vi "generate_DAC_voltages_V3_justFPGATrajectory.vi"(7 "focus mode?":bool, 8 "derived values":T1, 9 "scan specification":T4={"x amplitude"=0, "x resolution (pixels)"=0, "x offset fly-forward (iterations)"=0, "x offset fly-back (iterations)"=0, "y resolution (nr. of lines)"=0, "y step size"=0, "iterations per pixel"=0, "number of frames"=0, "y offset (pixels)"=0, "number of y-brake lines  (before y-fly-back)"=0, "number y-brake lines (after y-fly-back)"=0, "number of y-fly-back steps"=8, "lines per z step"=0, "number of z/intensity tuples"=0, "number of repetitions (volumes or planes)"=0, "z step size derived"=0, "choose the beginning of z scan"=FALSE, "number of frames (settings)"=0, "FPGA trajectory?"=FALSE}, 10 "counter cluster in":T2, 11 "resonant trigger":bool) -> (0 "acquire?":bool, 1 "fly-back acquisition phase?":bool, 2 "counter cluster out":T2, 3 "DAC voltages":T3 {"ch6" max=4095 step=1; "ch5" max=4095 step=1; "ch4" max=4095 step=1; "ch3" max=4095 step=1; "ch2" max=4095 step=1; "ch1" max=4095 step=1; "ch0" max=4095 step=1})   [LabVIEW 2010]
uses:
  scan_specification_cluster.ctl
  common_typedefs/DAC_voltage_cluster.ctl
  counter_cluster.ctl
  derived_values_cluster.ctl
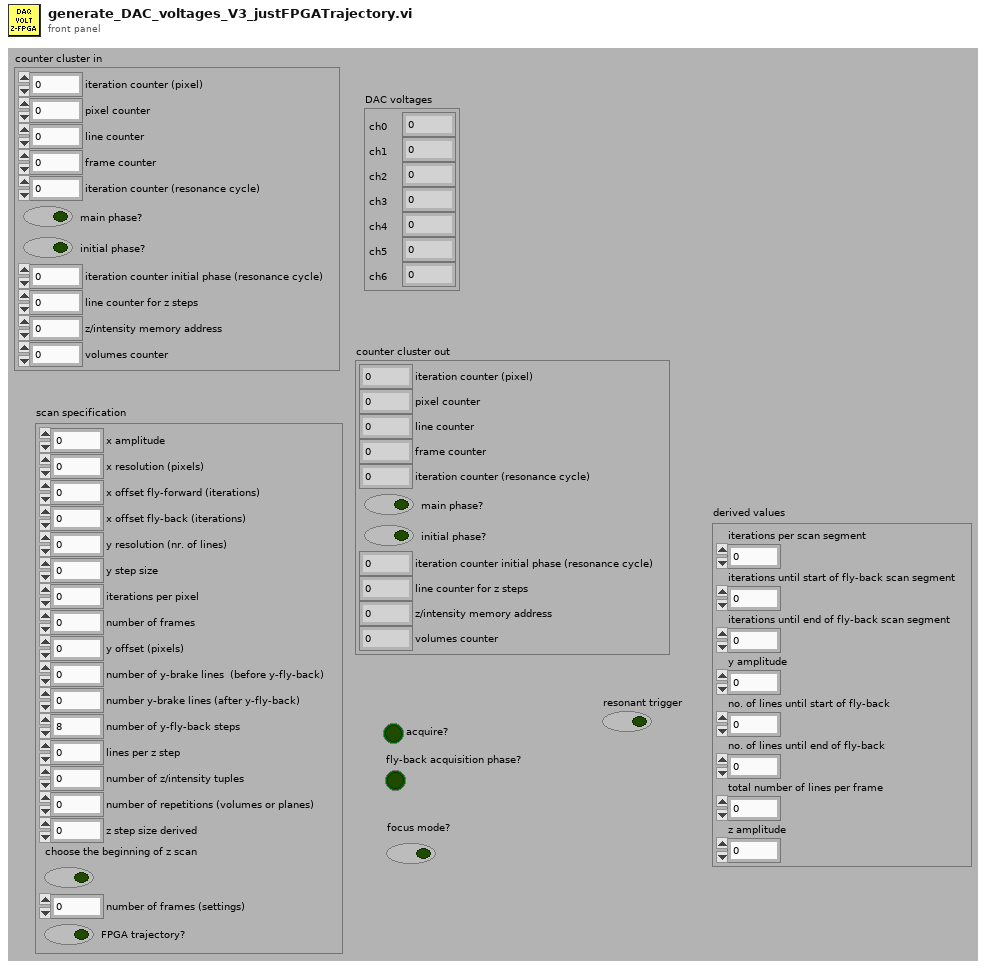
[diagram p1: front panel]
types:
  T1 = typedef "derived_values_cluster.ctl" = cluster{"iterations per scan segment":u16, "iterations until start of fly-back scan segment":u16, "iterations until end of fly-back scan segment":u16, "y amplitude":u16, "no. of lines until start of fly-back":u16, "no. of lines until end of fly-back":u16, "total number of lines per frame ":u16, "z amplitude":u16}
  T2 = typedef "counter_cluster.ctl" = cluster{"iteration counter (pixel)":u16, "pixel counter":u16, "line counter":u16, "frame counter":u16, "iteration counter (resonance cycle)":u16, "main phase?":bool, "initial phase?":bool, "iteration counter initial phase (resonance cycle)":u16, "line counter for z steps":u16, "z/intensity memory address":u32, "volumes counter":u16}
  T3 = typedef "DAC_voltage_cluster.ctl" = cluster{"ch0":u16, "ch1":i16, "ch2":i16, "ch3":u16, "ch4":u16, "ch5":u16, "ch6":u16}
  T4 = typedef "scan_specification_cluster.ctl" = cluster{"x amplitude":u16, "x resolution (pixels)":u16, "x offset fly-forward (iterations)":u16, "x offset fly-back (iterations)":u16, "y resolution (nr. of lines)":u16, "y step size":u16, "iterations per pixel":u16, "number of frames":i32, "y offset (pixels)":u16, "number of y-brake lines  (before y-fly-back)":u16, "number y-brake lines (after y-fly-back)":u16, "number of y-fly-back steps":u16, "lines per z step":u16, "number of z/intensity tuples":u16, "number of repetitions (volumes or planes)":i32, "z step size derived":u16, "choose the beginning of z scan":bool, "number of frames (settings)":i32, "FPGA trajectory?":bool}
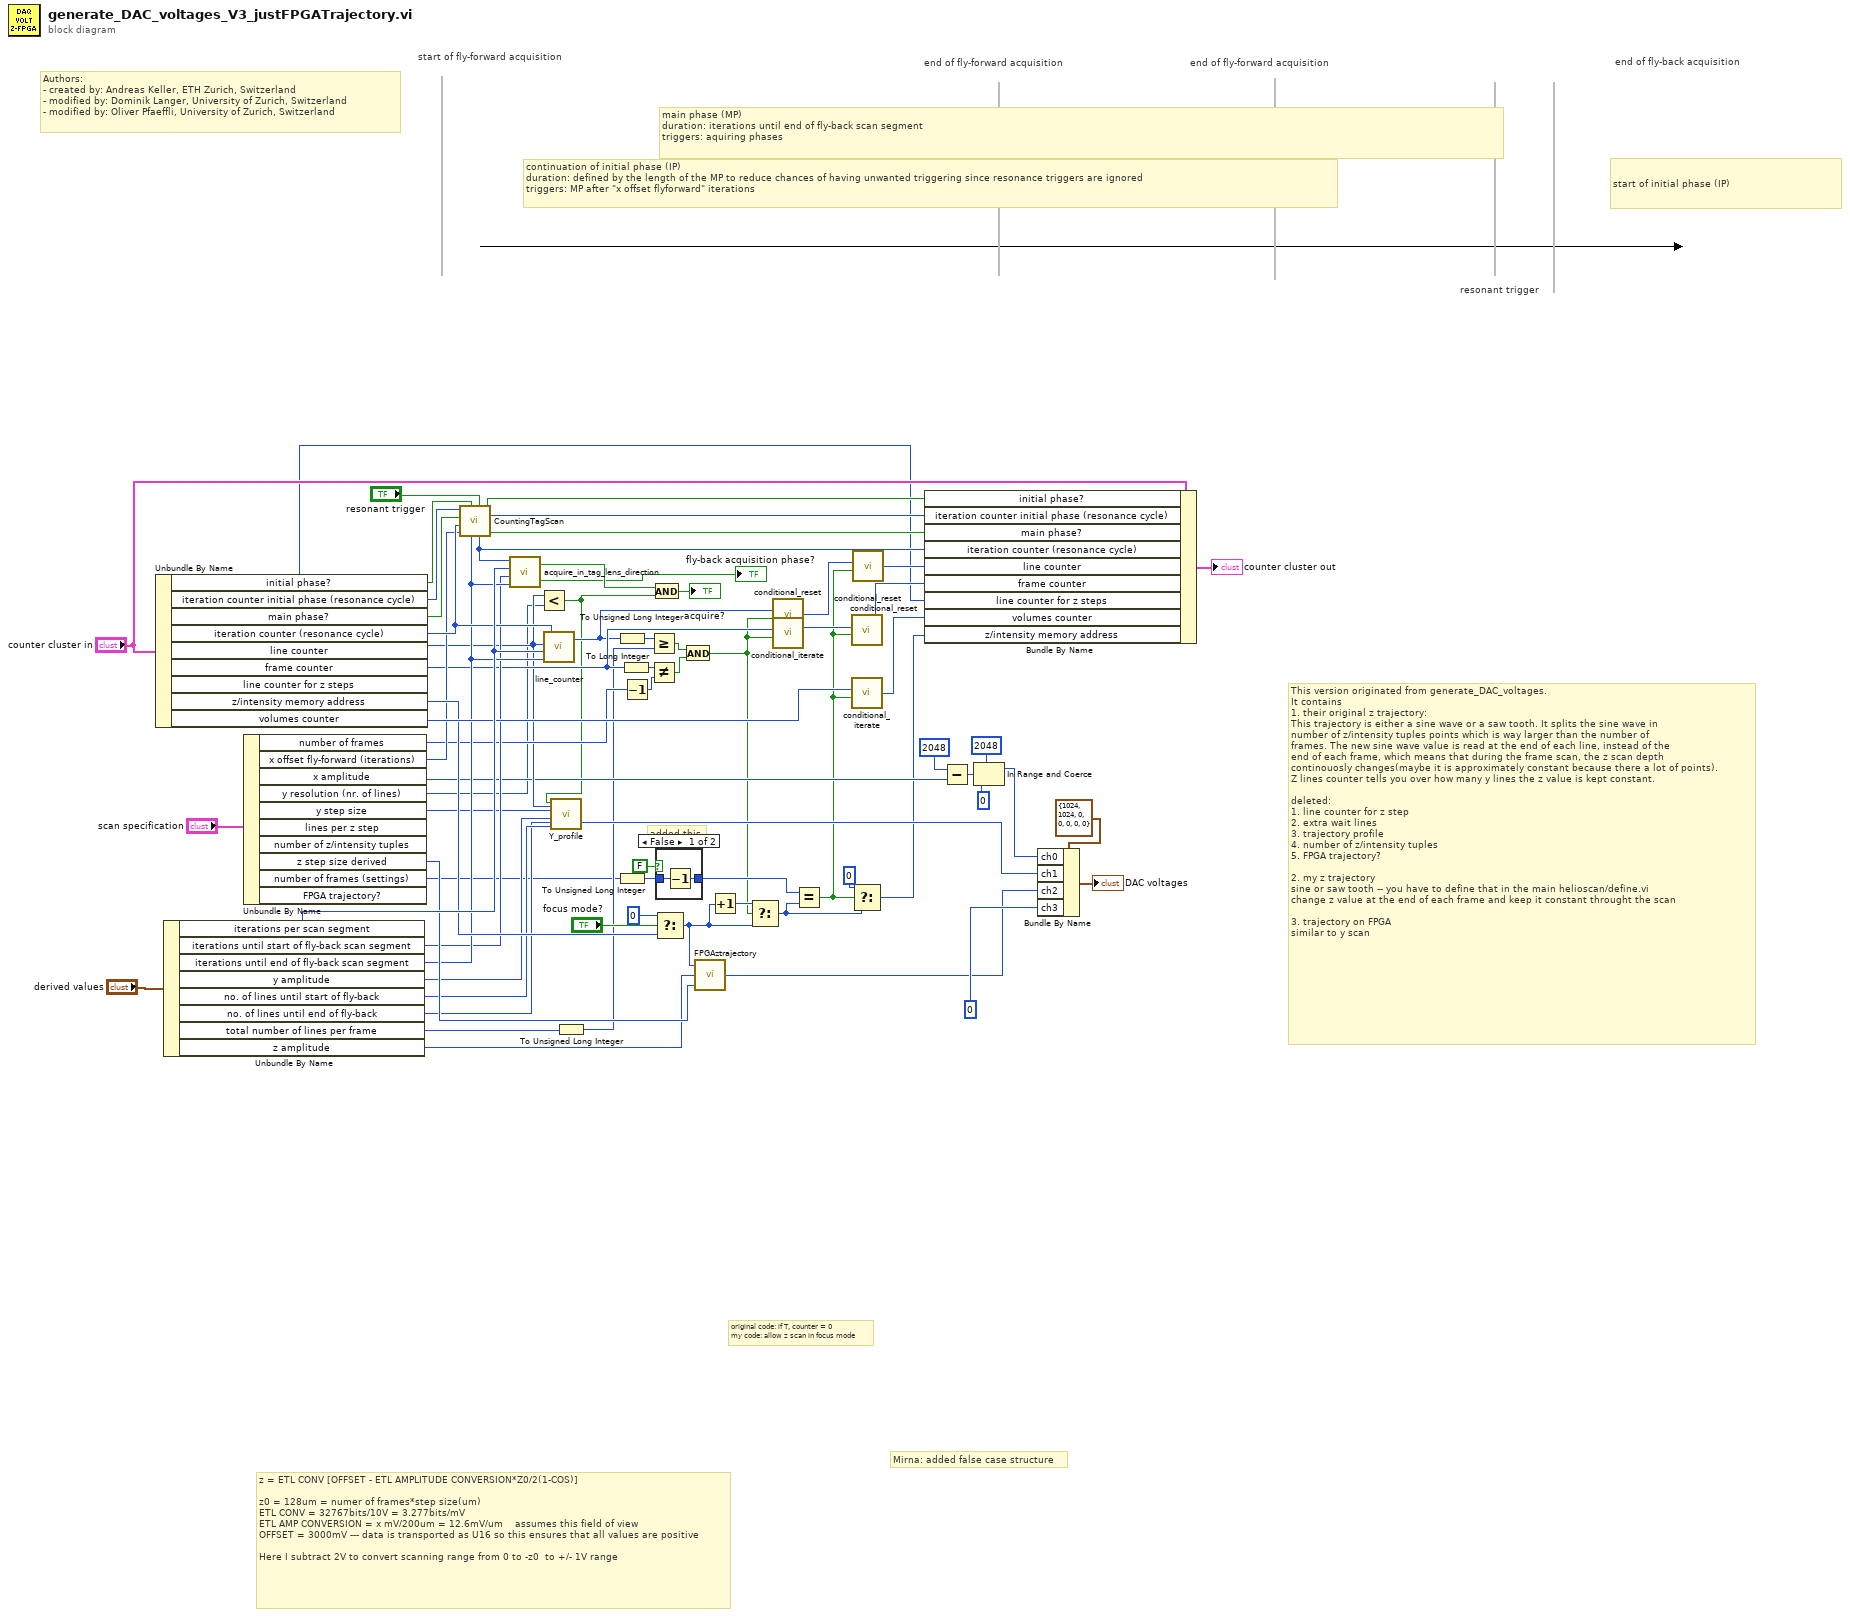
[diagram p0: block diagram]
diagram:
  # "This version originated from generate_DAC_voltages.\nIt contains \n1. their original z trajectory:\nThis trajectory is either a sine wave or a saw tooth. It splits the sine wave in\nnumber of z/intensity tuples points which is way larger than the number of\nframes. The new sine wave value is read at the end of each line, instead of the\nend of each frame, which means that during the frame scan, the z scan depth \ncontinouosly changes(maybe it is approximately constant because there a lot of points).\nZ lines counter tells you over how many y lines the z value is kept constant.\n\ndeleted: \n1. line counter for z step\n2. extra wait lines\n3. trajectory profile\n4. number of z/intensity tuples\n5. FPGA trajectory?\n\n2. my z trajectory\nsine or saw tooth -- you have to define that in the main helioscan/define.vi\nchange z value at the end of each frame and keep it constant throught the scan\n\n3. trajectory on FPGA\nsimilar to y scan"
  # "added this"
  # "z = ETL CONV [OFFSET - ETL AMPLITUDE CONVERSION*Z0/2(1-COS)]\n\nz0 = 128um = numer of frames*step size(um)\nETL CONV = 32767bits/10V = 3.277bits/mV\nETL AMP CONVERSION = x mV/200um = 12.6mV/um    assumes this field of view\nOFFSET = 3000mV --- data is transported as U16 so this ensures that all values are positive\n\nHere I subtract 2V to convert scanning range from 0 to -z0  to +/- 1V range"
  # "original code: if T, counter = 0\nmy code: allow z scan in focus mode"
  # "Mirna: added false case structure"
  # "start of initial phase (IP)"
  # "continuation of initial phase (IP)\nduration: defined by the length of the MP to reduce chances of having unwanted triggering since resonance triggers are ignored\ntriggers: MP after \"x offset flyforward\" iterations"
  # "end of fly-back acquisition"
  # "end of fly-forward acquisition"
  # "end of fly-forward acquisition"
  # "start of fly-forward acquisition"
  # "main phase (MP)\nduration: iterations until end of fly-back scan segment\ntriggers: aquiring phases"
  # "resonant trigger"
  # "Authors: \n- created by: Andreas Keller, ETH Zurich, Switzerland\n- modified by: Dominik Langer, University of Zurich, Switzerland\n- modified by: Oliver Pfaeffli, University of Zurich, Switzerland"
  n1 = Unbundle By Name("counter cluster in") -> ("initial phase?"=w60:bool, "iteration counter initial phase (resonance cycle)"=w30:u16, "main phase?"=w49:bool, "iteration counter (resonance cycle)"=w29:u16, "line counter"=w20:u16, "frame counter"=w21:u16, "line counter for z steps"=w6:u16, "z/intensity memory address"=w44:u32, "volumes counter"=w51:u16)
  n2 = Unbundle By Name("derived values") -> ("iterations per scan segment"=w59:u16, "iterations until start of fly-back scan segment"=w27:u16, "iterations until end of fly-back scan segment"=w28:u16, "y amplitude"=w34:u16, "no. of lines until start of fly-back"=w18:u16, "no. of lines until end of fly-back"=w17:u16, "total number of lines per frame"=w40:u16, "z amplitude"=w35:u16)
  n3 = Unbundle By Name("scan specification") -> ("number of frames"=w22:i32, "x offset fly-forward (iterations)"=w25:u16, "x amplitude"=w15:u16, "y resolution (nr. of lines)"=w1:u16, "y step size"=w19:u16, "z step size derived"=w41:u16, "number of frames (settings)"=w4:i32)  [unwired: 3 out]
  n4 = call "CountingTagScan.vi"("resonant trigger"="resonant trigger", "initial phase?"=w60, "iteration counter initial phase (resonance cycle)"=w30, "main phase?"=w49, "iterations until end of fly-back scan segment"=w28, "iteration counter (resonance cycle)"=w29, "x offset fly-forward (iterations)"=w25) -> ("initial phase? OUT"=w32:bool, "iteration counter initial phase (resonance cycle) out"=w31:u16, "main phase? OUT"=w24:bool, "iteration counter (resonance cycle) out"=w8:u16)
  n5 = call "acquire_in_tag_lens_direction.vi"("iterations until end of fly-back scan segment"=w28, "iterations until start of fly-back scan segment"=w27, "iterations per scan segment"=w59, "iteration counter (resonance cycle) out"=w8) -> ("flyback phase?"=→"fly-back acquisition phase?":bool, "acquire during flyforward or flyback phase?"=w62:bool)
  n6 = Less?(x=w20, y=w1) -> (x < y?=w11:bool)
  n7 = call "line_counter.vi"("iterations until end of fly-back scan segment"=w28, "iterations per scan segment"=w59, "line counter in"=w20, "iteration counter (resonance cycle)"=w29) -> ("line counter out"=w13:u16)  [unwired: 1 out]
  n8 = call "Y_profile.vi"("no. of lines until end of fly-back"=w17, "line counter"=w20, "no. of lines until start of fly-back"=w18, "y amplitude"=w34, "y step size"=w19, "true when line counter smaller than y resolution"=w11) -> ("y signal"=w48:i16)  [unwired: 1 in]
  n9 = To Unsigned Long Integer(number=w40) -> (unsigned 32bit integer=w5:u32)
  n10 = To Unsigned Long Integer(number=w13) -> (unsigned 32bit integer=w39:u32)
  n11 = To Unsigned Long Integer(number=w4) -> (unsigned 32bit integer=w57:u32)
  n12 = To Long Integer(number=w21) -> (32bit integer=w52:i32)
  n13 = Decrement(x=w22) -> (x-1=w53:i32)
  n14 = Greater Or Equal?(x=w39, y=w5) -> (x >= y?=w54:bool)
  n15 = Not Equal?(x=w52, y=w53) -> (x != y?=w16:bool)
  n16 = And(x=w62, y=w11) -> (x .and. y?=→"acquire?":bool)
  n17 = Select(t=u32 0, s="focus mode?", f=w44) -> (s? t:f=w45:u32)
  n18 = case shown="False" FALSE {
    tunnel: w57 -> [w73 w74]
    tunnel: [w72 w74] -> w38
    frame False {
      n19 = Decrement(x=w73) -> (x-1=w72:u32)
    }
    frame True {
    }
  }
  n20 = And(x=w54, y=w16) -> (x .and. y?=w3:bool)
  n21 = call "FPGAztrajectory.vi"("z step size derived"=w41, "z amplitude"=w35, "z/intensity memory address"=w45) -> ("Z trajectory"=w46:i16)
  n22 = Increment(x=w45) -> (x+1=w58:u32)
  n23 = Select(t=w58, s=w3, f=w45) -> (s? t:f=w9:u32)
  n24 = call "conditional_reset.vi"("reset?"=w3, "number in"=w13) -> ("number out"=w2:u16)  [unwired: 4 in]
  n25 = call "conditional_iterate.vi"("iterate?"=w3, "number in"=w21) -> ("number out"=w42:u16)  [unwired: 4 in]
  n26 = Equal?(x=w38, y=w9) -> (x = y?=w7:bool)
  n27 = call "conditional_reset.vi"("reset?"=w7, "number in"=w42) -> ("number out"=w43:u16)  [unwired: 4 in]
  n28 = call "conditional_iterate.vi"("iterate?"=w7, "number in"=w51) -> ("number out"=w56:u16)  [unwired: 4 in]
  n29 = Select(t=u32 0, s=w7, f=w9) -> (s? t:f=w10:u32)
  n30 = call "conditional_reset.vi"("reset?"=w7, "number in"=w2) -> ("number out"=w55:u16)  [unwired: 4 in]
  n31 = Bundle By Name(cluster="counter cluster in", "initial phase?"=w32, "iteration counter initial phase (resonance cycle)"=w31, "main phase?"=w24, "iteration counter (resonance cycle)"=w8, "line counter"=w55, "frame counter"=w43, "line counter for z steps"=w6, "volumes counter"=w56, "z/intensity memory address"=w10) -> (→"counter cluster out":T2)
  n32 = Subtract(x=u16 2048, y=w15) -> (x-y=w66:u16)
  n33 = In Range and Coerce(upper limit=u16 2048, x=w66, lower limit=u16 0) -> (coerced(x)=w65:u16)  [unwired: 1 out]
  n34 = Bundle By Name(cluster=T3 {"ch0"=1024, "ch1"=1024, "ch2"=0, "ch3"=0, "ch4"=0, "ch5"=0, "ch6"=0} ("DAC voltage"), "ch0"=w65, "ch1"=w48, "ch2"=w46, "ch3"=u16 0 ("intensity")) -> (→"DAC voltages":T3)
